vi "Set Frequency.vi"(8 "error in (no error)":errorcluster, 10 "frequency (Hz)":dbl, 11 "General Hardware in":refnum<class "General Hardware.lvclass">) -> (0 "error out":errorcluster, 3 "General Hardware out":refnum<class "General Hardware.lvclass">)   [LabVIEW 2020, in "General Hardware.lvclass"]
uses:
  General Hardware.lvclass
  General Hardware.lvclass/General Hardware.ctl
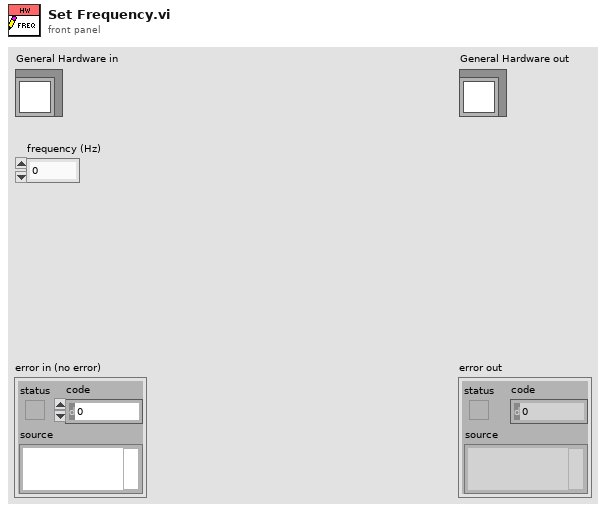
[diagram p1: front panel]
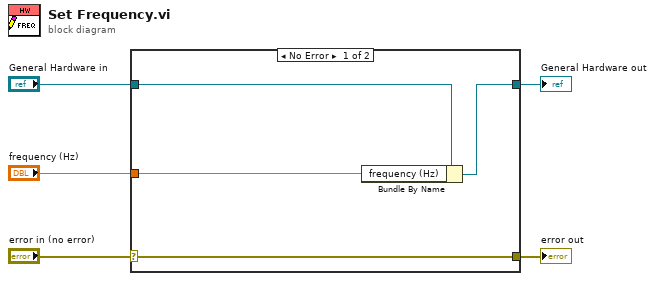
[diagram p0: block diagram]
diagram:
  n1 = case shown="No Error" "error in (no error)" {
    selector: "error in (no error)" -> [w9 w10]
    tunnel: [w9 w10] -> w4
    tunnel: [w7 w11] -> w2
    tunnel: "General Hardware in" -> [w8 w11]
    tunnel: "frequency (Hz)" -> [w6 _]
    frame No Error {
      n2 = Bundle By Name(cluster=w8, "frequency (Hz)"=w6) -> (w7:refnum<class "General Hardware.lvclass">)
    }
    frame Error {
    }
  }
  "error out" <- w4
  "General Hardware out" <- w2
